vi "SteeringValidate - second.vi"() -> ()   [LabVIEW 2016]
uses:
  <vilib>/Platform/TimedLoop/XDataNode/timing_clust.ctl
  <vilib>/Platform/TimedLoop/XDataNode/nitl_modes.ctl
  <vilib>/Platform/TimedLoop/XDataNode/wakeup.ctl
  <vilib>/FPGAPlugInAG/roboRIO/niLvFpga_Open_roboRIO.vi
  <vilib>/rvi/interface/common/dynamic/niFpgaDynamicAddResources.vi
  <vilib>/FPGAPlugInAG/Dynamic/niLvFpga_Reset_Dynamic.vi
  <vilib>/FPGAPlugInAG/Dynamic/niLvFpga_Run_Dynamic.vi
  <vilib>/Utility/error.llb/Error Cluster From Error Code.vi
  <vilib>/rvi/errors/niLvFpgaAdjustHostInterfaceError.vi
  <vilib>/FPGAPlugInAG/Dynamic/niLvFpga_Abort_Dynamic.vi
  <vilib>/FPGAPlugInAG/Dynamic/niLvFpga_Close_Dynamic.vi
  <vilib>/rvi/interface/nirviOpenFPGA/nirviOpenFPGA.xnode
  FPGA Bitfiles/AutoBikeProject_FPGATarget_FPGASteeringVali_0ktHJXMggMw.lvbitx
  <vilib>/rvi/interface/nirviMethod/nirviMethod.xnode
  <vilib>/Platform/TimedLoop/XDataNode/XDataNode.xnode
  <vilib>/rvi/interface/nirviReadWriteControl/nirviReadWriteControl.xnode
  <vilib>/rvi/interface/nirviCloseFPGA/nirviCloseFPGA.xnode
  <vilib>/Platform/TimedLoop/XDataNode/XDNodeRunTimeDep.lvlib
  <vilib>/rvi/interface/Simulation/niFpgaSimulationCallBeginRW.vi
  NiFpgaLv.dll
panel:
  in  "Frequency of duty cycle 2":u32=40000
  out "duty cycle":dbl
  in  "Reset steering angle":bool
  out "Finished Late? [i-1]":bool
  in  "Stop":bool
  in  "Frequency of duty cycle":u32=40000
  in  "Direction":bool
  out "error out":errorcluster
  in  "error in (no error)":errorcluster
  # "Newton"
  # "Pulstid"
  # "DC"
  # "0.0\n0.05\n0.1\n0.15\n0.2\n0.25\n0.3\n0.35\n0.4\n0.45\n0.5\n0.55\n0.6\n0.65\n0.7\n0.75\n0.8\n0.85\n0.9"
  # "Front Panel Controls"
  # "CC"
  # "CW"
  # "100 = 0.2s\n200 = 0.4s\n300 = 0.6s\n400 = 0.8s\n500 = 1.0s"
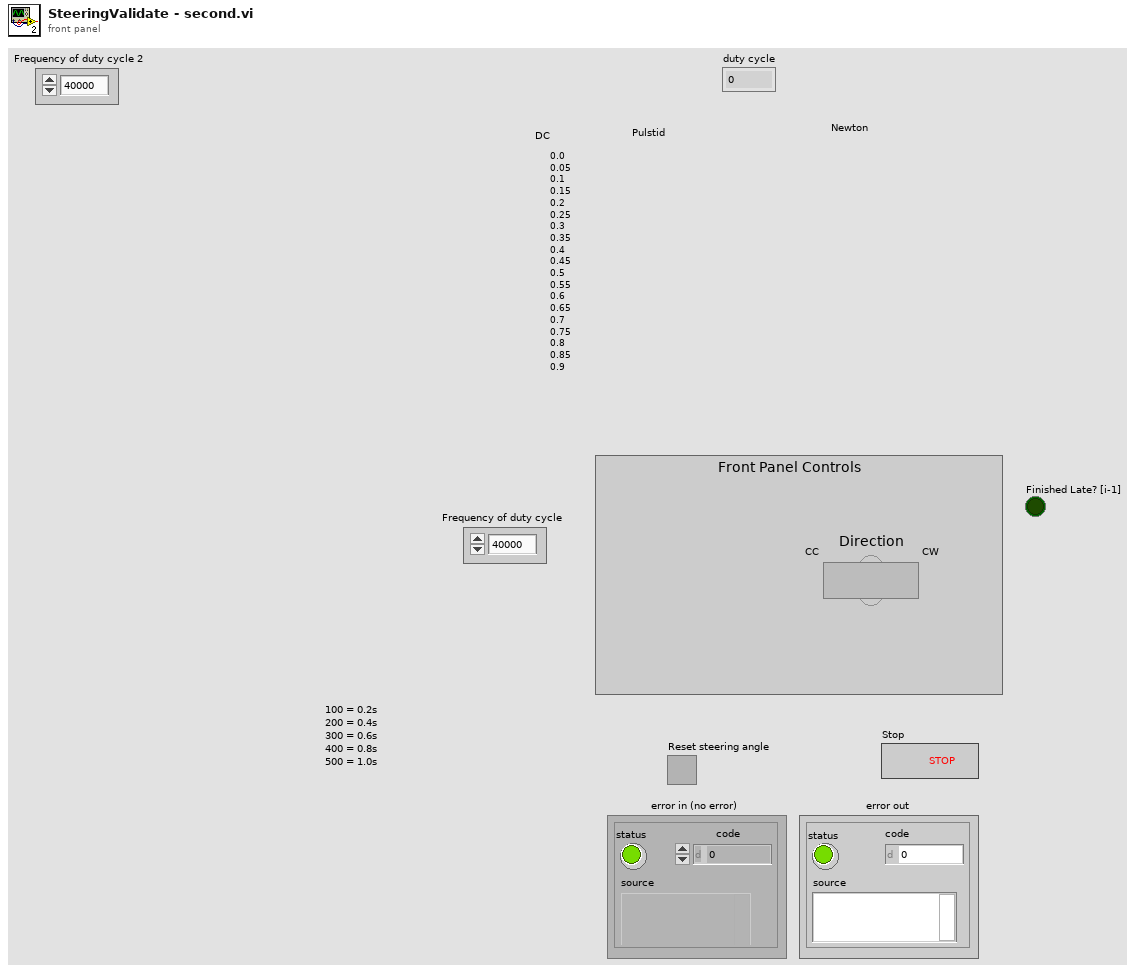
[diagram p1: front panel]
types:
  T1 = enum16{"open", "open or create", "create or replace", "create", "open (read-only)"}
  T2 = typedef "XDNodeRunTimeDep.lvlib/timing_clust.ctl" = cluster{"Expected End [f-1]":u64, "Actual End [f-1]":u64, "Finished Late? [f-1]":bool, "Expected End [i-1]":u64, "Actual End [i-1]":u64, "Finished Late? [i-1]":bool, "Expected Start [i]":u64, "Actual Start [i]":u64, "Expected Start [f]":u64, "Actual Start [f]":u64, "Source Name":string, "Structure Name":string, "Period":i64, "Deadline":i64, "Offset":i64, "Start":i64, "Priority":i32, "Timeout":i32, "Mode":T3, "Wakeup Reason":T4, "Error":errorcluster, "Source Type":string, "Secondary Source Type":string, "Global End Time":u64, "Global Start Time":u64, "Frame Duration":u64, "Iteration Duration":u64, "Assigned CPU":i32, "I/O Scan Engine Mode":u32}
  T3 = typedef "XDNodeRunTimeDep.lvlib/nitl_modes.ctl" = enum32{"No Change", "Process missed periods, maintain original phase", "Discard missed periods, maintain original phase", "Process missed periods, ignore original phase", "Discard missed periods, ignore original phase"}
  T4 = typedef "XDNodeRunTimeDep.lvlib/wakeup.ctl" = enum32{"Normal", "Aborted", "Asynchronous wakeup", "Timing source error", "Timed loop error", "Timeout"}
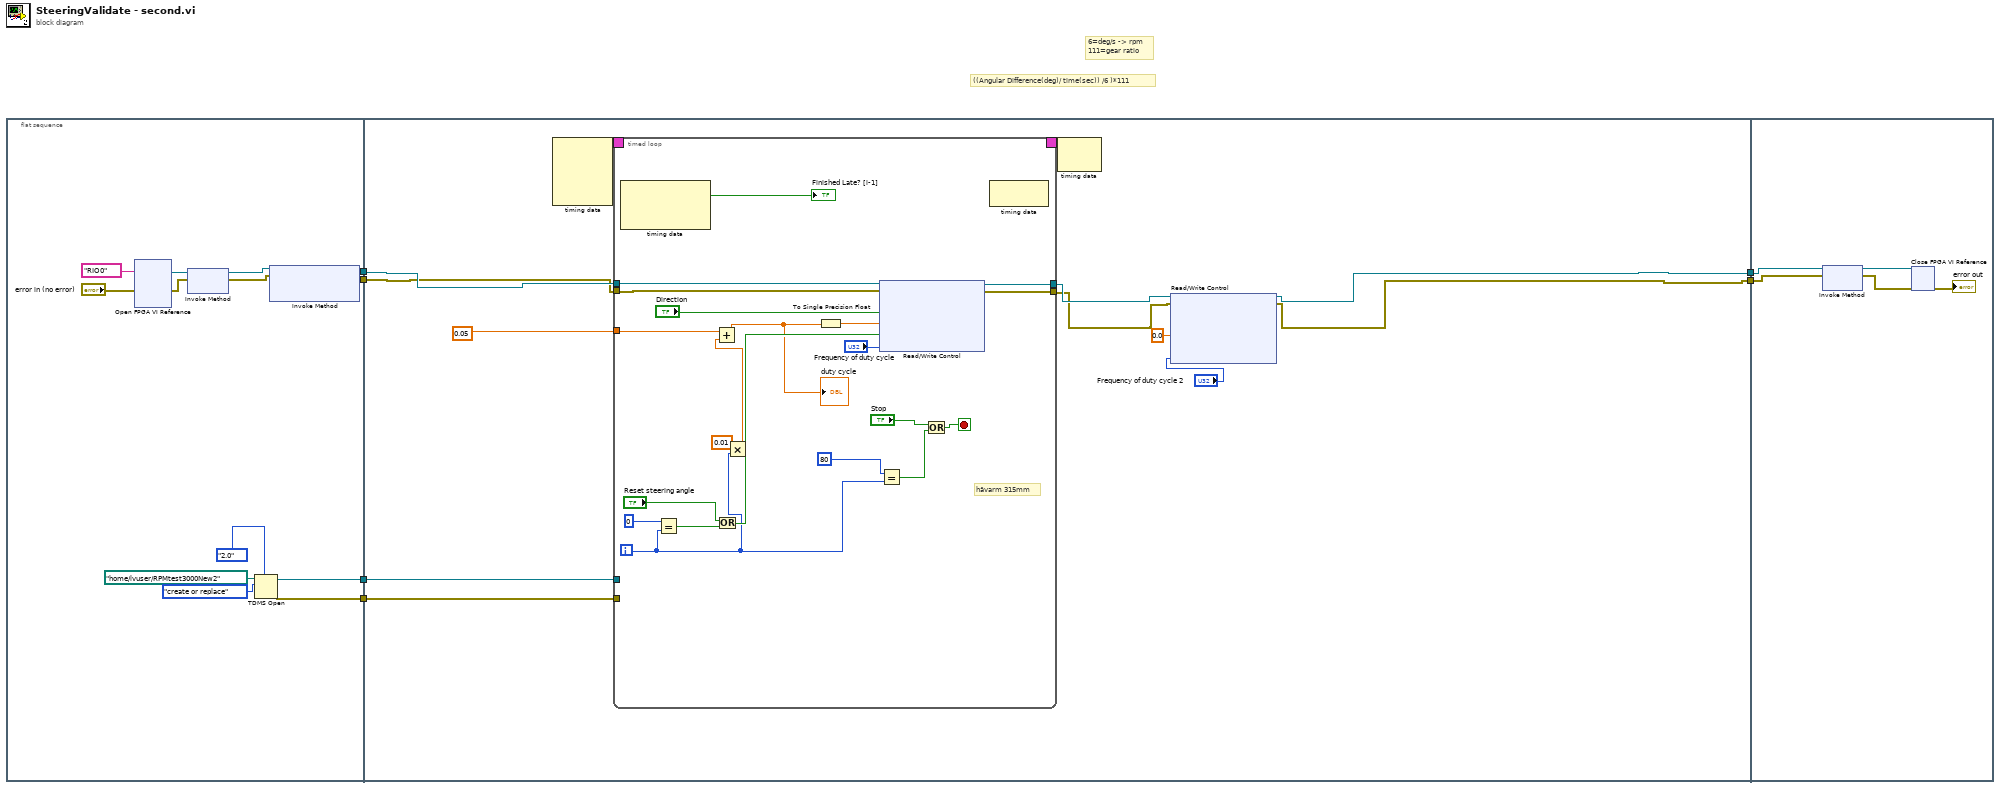
[diagram p0: block diagram]
diagram:
  # "6=deg/s -> rpm\n111=gear ratio"
  # "((Angular Difference(deg)/ time(sec)) /6 )*111"
  n1 = flat-sequence {
    tunnel: [w10] -> w6
    tunnel: [w9] -> w5
    tunnel: [w12] -> w4
    tunnel: [w11] -> w3
    tunnel: w6 -> [w29]
    tunnel: w5 -> [w28]
    tunnel: w4 -> [w31]
    tunnel: w3 -> [w30]
    tunnel: [w32] -> w2
    tunnel: [w27] -> w1
    tunnel: w2 -> [w60]
    tunnel: w1 -> [w59]
    frame #0 {
      n2 = xnode "Open FPGA VI Reference"("error in"="error in (no error)", "resource name"=tag "RIO0") -> ("FPGA VI Reference Out"=w17:refnum<k20>, "error out"=w16:errorcluster)
      n3 = xnode "Invoke Method"("FPGA VI Reference In"=w17, "error in"=w16) -> ("FPGA VI Reference Out"=w7:refnum<k20>, "error out"=w8:errorcluster)
      n4 = TDMS Open(7:enum16{"1.0", "2.0"}."2.0" ("file format version (2.0)"), 10:T1."create or replace" ("operation (0:open)"), 11:path "/home/lvuser/RPMtest3000New2" ("file path")) -> (0:w11:errorcluster, 3:w12:refnum<k34>)  [unwired: 4 in]
      n5 = xnode "Invoke Method"("FPGA VI Reference In"=w7, "error in"=w8) -> ("FPGA VI Reference Out"=w10:refnum<k20>, "error out"=w9:errorcluster)  [unwired: 1 in]
    }
    frame #1 {
      n6 = node-c288() -> (w26:T2)  [unwired: 4 in]
      n7 = timed-loop {
        timing: w26 -> [_]
        timing-out: [_] -> w25
        tunnel: [w47] -> w24
        tunnel: [w46] -> w23
        tunnel: w29 -> [w53]
        tunnel: w28 -> [w52]
        tunnel: w31 -> [_]
        tunnel: w30 -> [_]
        tunnel: 0.05 -> [w35]
        i -> [w36]
        stop <- w41 stop-if-true
        # "hävarm 315mm"
        n8 = node-c288() -> (→"Finished Late? [i-1]":bool)  [unwired: 1 in, 2 out]
        n9 = Equal?(x=0, y=w36) -> (x = y?=w44:bool)
        n10 = Or(x="Reset steering angle", y=w44) -> (x .or. y?=w43:bool)
        n11 = Multiply(x=0.01, y=w36) -> (x*y=w34:dbl)
        n12 = Add(x=w35, y=w34) -> (x+y=w33:dbl)
        "duty cycle" <- w33
        n13 = To Single Precision Float(number=w33) -> (single precision float=w49:sgl)
        n14 = xnode "Read/Write Control"("FPGA VI Reference In"=w53, "error in"=w52, "Direction"="Direction", "Front Panel Duty Cycle"=w49, "Reset counter"=w43, "Freq"="Frequency of duty cycle") -> ("FPGA VI Reference Out"=w47:refnum<k20>, "error out"=w46:errorcluster)  [unwired: 1 out]
        n15 = Equal?(x=80, y=w36) -> (x = y?=w38:bool)
        n16 = Or(x="Stop", y=w38) -> (x .or. y?=w41:bool)
        n17 = node-c288() -> ()  [unwired: 1 in, 1 out]
      }
      n18 = node-c288(w25) -> ()  [unwired: 1 out]
      n19 = xnode "Read/Write Control"("FPGA VI Reference In"=w24, "error in"=w23, "Front Panel Duty Cycle"=sgl 0.0, "Freq"="Frequency of duty cycle 2") -> ("FPGA VI Reference Out"=w32:refnum<k20>, "error out"=w27:errorcluster)  [unwired: 2 in, 1 out]
    }
    frame #2 {
      n20 = xnode "Invoke Method"("FPGA VI Reference In"=w60, "error in"=w59) -> ("FPGA VI Reference Out"=w62:refnum<k20>, "error out"=w63:errorcluster)
      n21 = xnode "Close FPGA VI Reference"("FPGA VI Reference In"=w62, "error in"=w63) -> ("error out"=→"error out":errorcluster)
    }
  }
